vi "Prepare IFDs.vi"(8 "error in (no error)":errorcluster, 11 "TIFF in":refnum<class "TIFF.lvclass">) -> (0 "error out":errorcluster, 3 "TIFF out":refnum<class "TIFF.lvclass">)   [LabVIEW 2018, in "BinaryTIFF.lvlib" / "TIFF.lvclass"]
uses:
  TIFF.lvclass
  TIFF.lvclass/TIFF.ctl
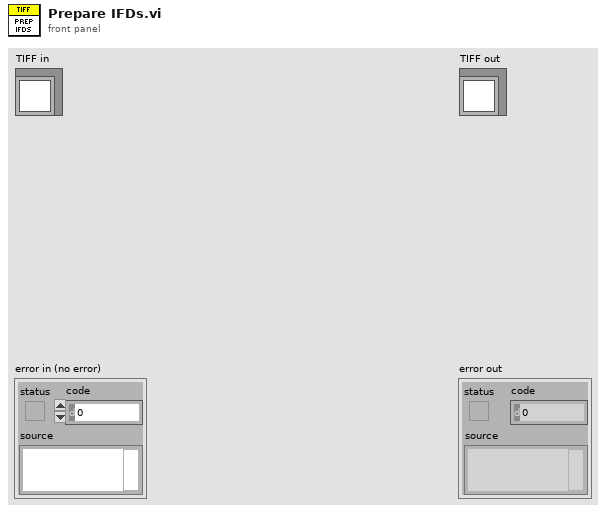
[diagram p1: front panel]
types:
  T1 = cluster{"Offset":u64, "Number of Entries":u64, "IFD Entries":cluster{"Tag":u16, "Data Type":u16, "Number of Elements":u64, "Data":variant}[]}
  T2 = cluster{"Tag":u16, "Data Type":u16, "Number of Elements":u64, "Data":variant}
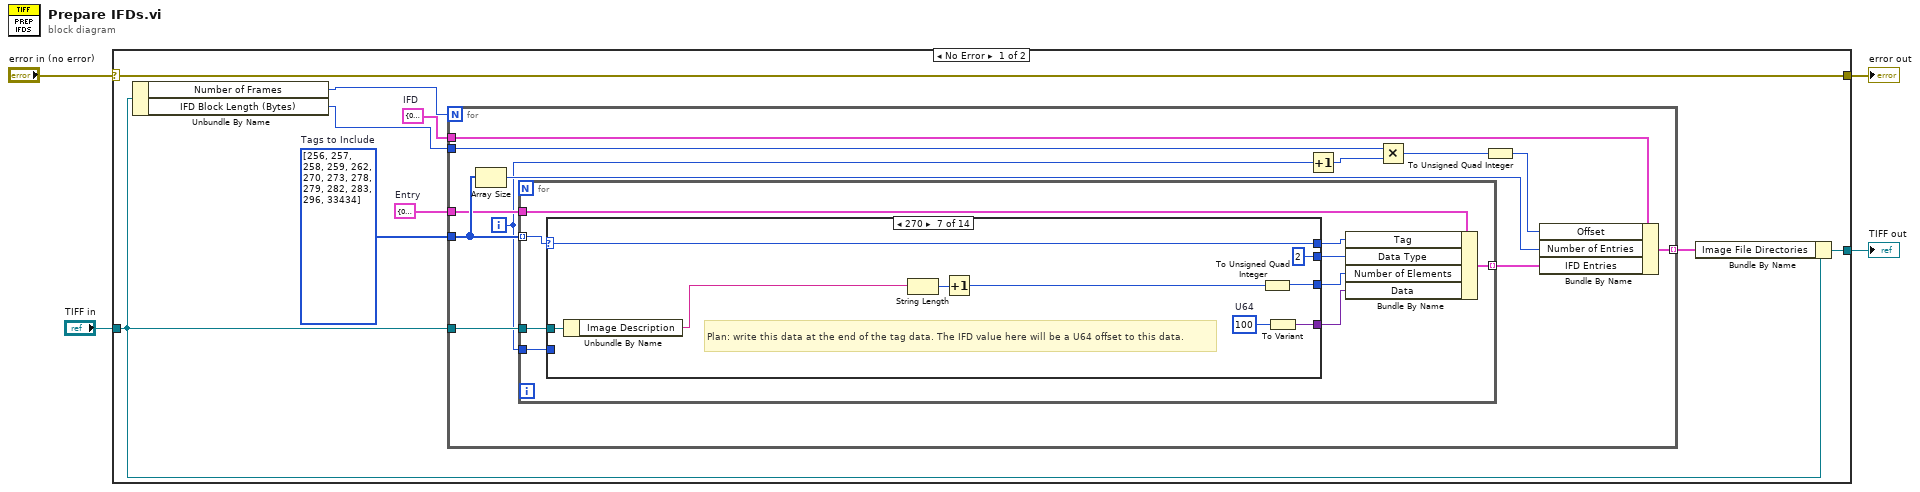
[diagram p0: block diagram]
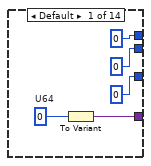
[diagram p2: hidden frame]
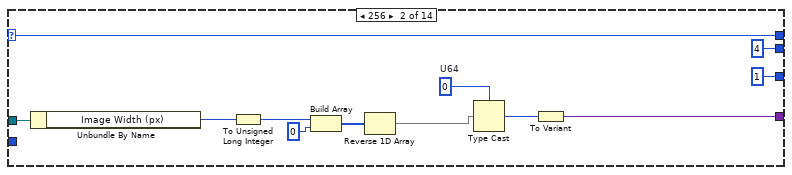
[diagram p3: hidden frame]
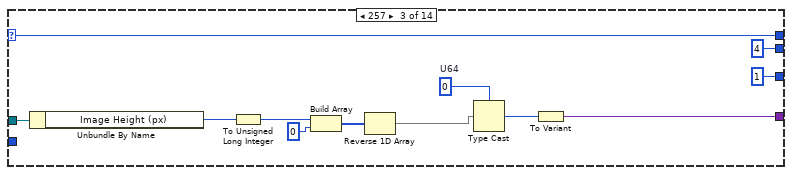
[diagram p4: hidden frame]
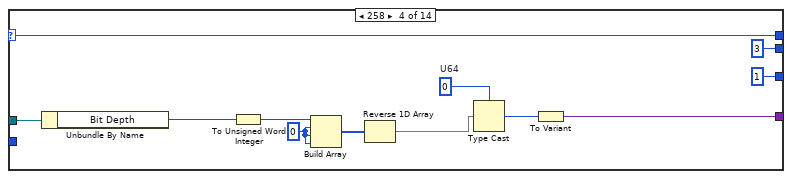
[diagram p5: hidden frame]
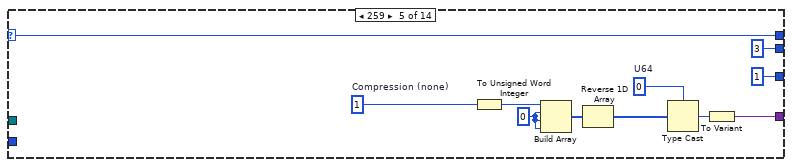
[diagram p6: hidden frame]
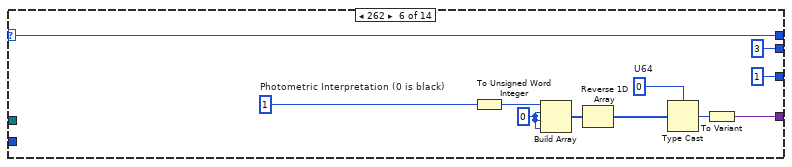
[diagram p7: hidden frame]
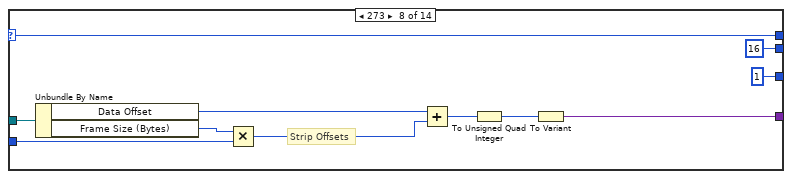
[diagram p8: hidden frame]
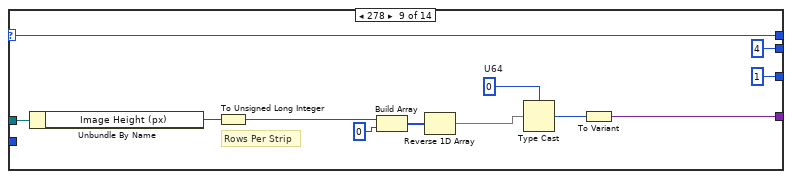
[diagram p9: hidden frame]
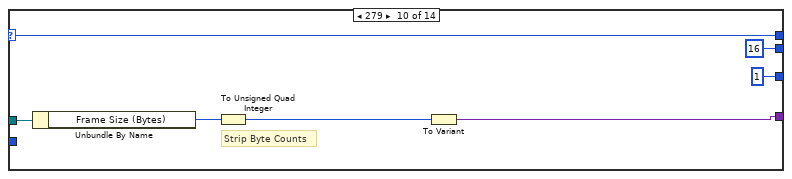
[diagram p10: hidden frame]
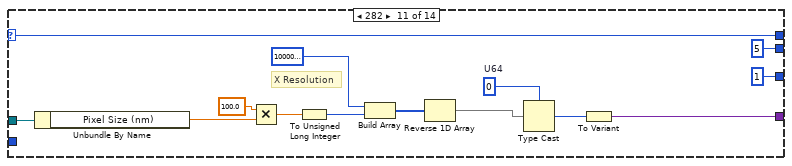
[diagram p11: hidden frame]
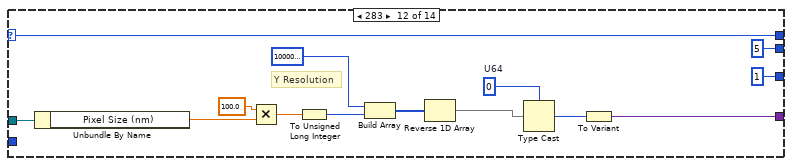
[diagram p12: hidden frame]
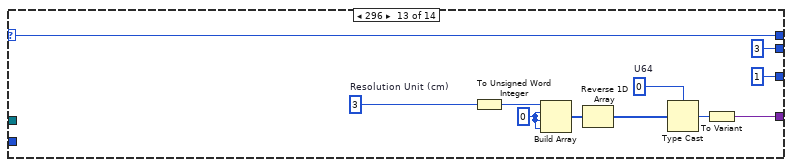
[diagram p13: hidden frame]
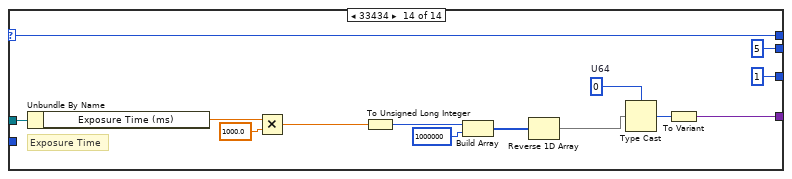
[diagram p14: hidden frame]
diagram:
  n1 = case shown="No Error" "error in (no error)" {
    selector: "error in (no error)" -> [w13 w191]
    tunnel: [w13 w191] -> w3
    tunnel: [w10 w190] -> w1
    tunnel: "TIFF in" -> [w8 w190]
    frame No Error {
      w6 = T1 {"Offset"=0, "Number of Entries"=0, "IFD Entries"=[]}  # IFD
      w7 = T2 {"Tag"=0, "Data Type"=0, "Number of Elements"=0, "Data"=variant}  # Entry
      w11 = u16[] [256, 257, 258, 259, 262, 270, 273, 278, 279, 282, 283, 296, 33434]  # Tags to Include
      n2 = Unbundle By Name(w8) -> ("Number of Frames"=w12:u32, "IFD Block Length (Bytes)"=w9:u32)
      n3 = for {
        N: w12 -> [_]
        tunnel: w11 -> [w22]
        tunnel: w9 -> [w25]
        tunnel: w6 -> [w24]
        tunnel: [w20] -> w5 mode=indexing
        tunnel: w7 -> [w19]
        tunnel: w8 -> [w18]
        i -> [w14]
        n4 = Array Size(array=w22) -> (size(s)=w23:i32)
        n5 = for {
          tunnel: w22 -> [w34] mode=indexing
          tunnel: w18 -> [w33]
          tunnel: w19 -> [w32]
          tunnel: [w31] -> w15 mode=indexing
          tunnel: w14 -> [w26]
          n6 = case shown="270" w34 {
            selector: w34 -> [_ w50 w62 w74 w86 w97 w106 w117 w128 w135 w149 w163 w175 w189]
            tunnel: w33 -> [_ w51 w63 w75 _ _ w104 w114 w129 w136 w150 w164 _ w186]
            tunnel: [u16 0 ("Tag") w50 w62 w74 w86 w97 w106 w117 w128 w135 w149 w163 w175 w189] -> w30
            tunnel: [u16 0 ("Data Type") u16 4 ("Data Type") u16 4 ("Data Type") u16 3 ("Data Type") u16 3 ("Data Type") u16 3 ("Data Type") u16 2 ("Data Type") u16 16 ("Data Type") u16 4 ("Data Type") u16 16 ("Data Type") u16 5 ("Data Type") u16 5 ("Data Type") u16 3 ("Data Type") u16 5 ("Data Type")] -> w29
            tunnel: [u64 0 ("Number of Elements") u64 1 ("Number of Elements") u64 1 ("Number of Elements") u64 1 ("Number of Elements") u64 1 ("Number of Elements") u64 1 ("Number of Elements") w102 u64 1 ("Number of Elements") u64 1 ("Number of Elements") u64 1 ("Number of Elements") u64 1 ("Number of Elements") u64 1 ("Number of Elements") u64 1 ("Number of Elements") u64 1 ("Number of Elements")] -> w28
            tunnel: w26 -> [_ _ _ _ _ _ _ w111 _ _ _ _ _ _]
            tunnel: [w35 w46 w58 w70 w82 w93 w103 w107 w124 w131 w143 w157 w172 w182] -> w27
            frame Default {
              w36 = u64 0  # U64
              n7 = To Variant(anything=w36) -> (Variant=w35:variant)
            }
            frame 256 {
              w43 = u64 0  # U64
              n8 = Unbundle By Name(w51) -> ("Image Width (px)"=w47:u32)
              n9 = To Unsigned Long Integer(number=w47) -> (unsigned 32bit integer=w45:u32)
              n10 = Build Array(w45, u32 0 ("element")) -> (w42:u32[])
              n11 = Reverse 1D Array(array=w42) -> (reversed array=w40:u32[])
              n12 = Type Cast(type=w43, x=w40) -> (*(type *) &x=w41:u64)
              n13 = To Variant(anything=w41) -> (Variant=w46:variant)
            }
            frame 257 {
              w55 = u64 0  # U64
              n14 = Unbundle By Name(w63) -> ("Image Height (px)"=w59:u32)
              n15 = To Unsigned Long Integer(number=w59) -> (unsigned 32bit integer=w56:u32)
              n16 = Build Array(w56, u32 0 ("element")) -> (w54:u32[])
              n17 = Reverse 1D Array(array=w54) -> (reversed array=w52:u32[])
              n18 = Type Cast(type=w55, x=w52) -> (*(type *) &x=w53:u64)
              n19 = To Variant(anything=w53) -> (Variant=w58:variant)
            }
            frame 258 {
              w67 = u64 0  # U64
              w68 = u16 0 ("element")
              n20 = Unbundle By Name(w75) -> ("Bit Depth"=w71:u32)
              n21 = To Unsigned Word Integer(number=w71) -> (unsigned 16bit integer=w69:u16)
              n22 = Build Array(w69, w68, w68, w68) -> (w66:u16[])
              n23 = Reverse 1D Array(array=w66) -> (reversed array=w64:u16[])
              n24 = Type Cast(type=w67, x=w64) -> (*(type *) &x=w65:u64)
              n25 = To Variant(anything=w65) -> (Variant=w70:variant)
            }
            frame 259 {
              w79 = u64 0  # U64
              w81 = u16 0 ("element")
              w83 = u64 1  # Compression (none)
              n26 = To Unsigned Word Integer(number=w83) -> (unsigned 16bit integer=w80:u16)
              n27 = Build Array(w80, w81, w81, w81) -> (w78:u16[])
              n28 = Reverse 1D Array(array=w78) -> (reversed array=w76:u16[])
              n29 = Type Cast(type=w79, x=w76) -> (*(type *) &x=w77:u64)
              n30 = To Variant(anything=w77) -> (Variant=w82:variant)
            }
            frame 262 {
              w90 = u64 0  # U64
              w92 = u16 0 ("element")
              w94 = u64 1  # Photometric Interpretation (0 is black)
              n31 = To Unsigned Word Integer(number=w94) -> (unsigned 16bit integer=w91:u16)
              n32 = Build Array(w91, w92, w92, w92) -> (w89:u16[])
              n33 = Reverse 1D Array(array=w89) -> (reversed array=w87:u16[])
              n34 = Type Cast(type=w90, x=w87) -> (*(type *) &x=w88:u64)
              n35 = To Variant(anything=w88) -> (Variant=w93:variant)
            }
            frame 270 {
              w101 = u64 100  # U64
              # "Plan: write this data at the end of the tag data. The IFD value here will be a U64 offset to this data."
              n36 = Unbundle By Name(w104) -> ("Image Description"=w98:string)
              n37 = String Length(string=w98) -> (length=w100:i32)
              n38 = Increment(x=w100) -> (x+1=w99:i32)
              n39 = To Unsigned Quad Integer(1:w99) -> (0:w102:u64)
              n40 = To Variant(anything=w101) -> (Variant=w103:variant)
            }
            frame 273 {
              # "Strip Offsets"
              n41 = Unbundle By Name(w114) -> ("Data Offset"=w113:u64, "Frame Size (Bytes)"=w112:u64)
              n42 = Multiply(x=w112, y=w111) -> (x*y=w110:u64)
              n43 = Add(x=w113, y=w110) -> (x+y=w109:u64)
              n44 = To Unsigned Quad Integer(1:w109) -> (0:w108:u64)
              n45 = To Variant(anything=w108) -> (Variant=w107:variant)
            }
            frame 278 {
              w121 = u64 0  # U64
              # "Rows Per Strip"
              n46 = Unbundle By Name(w129) -> ("Image Height (px)"=w125:u32)
              n47 = To Unsigned Long Integer(number=w125) -> (unsigned 32bit integer=w122:u32)
              n48 = Build Array(w122, u32 0 ("element")) -> (w120:u32[])
              n49 = Reverse 1D Array(array=w120) -> (reversed array=w118:u32[])
              n50 = Type Cast(type=w121, x=w118) -> (*(type *) &x=w119:u64)
              n51 = To Variant(anything=w119) -> (Variant=w124:variant)
            }
            frame 279 {
              # "Strip Byte Counts"
              n52 = Unbundle By Name(w136) -> ("Frame Size (Bytes)"=w132:u64)
              n53 = To Unsigned Quad Integer(1:w132) -> (0:w130:u64)
              n54 = To Variant(anything=w130) -> (Variant=w131:variant)
            }
            frame 282 {
              w142 = u64 0  # U64
              # "X Resolution"
              n55 = Unbundle By Name(w150) -> ("Pixel Size (nm)"=w146:dbl)
              n56 = Multiply(x=100.0, y=w146) -> (x*y=w144:dbl)
              n57 = To Unsigned Long Integer(number=w144) -> (unsigned 32bit integer=w138:u32)
              n58 = Build Array(u32 1000000000 ("element"), w138) -> (w141:u32[])
              n59 = Reverse 1D Array(array=w141) -> (reversed array=w137:u32[])
              n60 = Type Cast(type=w142, x=w137) -> (*(type *) &x=w140:u64)
              n61 = To Variant(anything=w140) -> (Variant=w143:variant)
            }
            frame 283 {
              w156 = u64 0  # U64
              # "Y Resolution"
              n62 = Unbundle By Name(w164) -> ("Pixel Size (nm)"=w160:dbl)
              n63 = Multiply(x=100.0, y=w160) -> (x*y=w158:dbl)
              n64 = To Unsigned Long Integer(number=w158) -> (unsigned 32bit integer=w153:u32)
              n65 = Build Array(u32 1000000000 ("element"), w153) -> (w155:u32[])
              n66 = Reverse 1D Array(array=w155) -> (reversed array=w151:u32[])
              n67 = Type Cast(type=w156, x=w151) -> (*(type *) &x=w154:u64)
              n68 = To Variant(anything=w154) -> (Variant=w157:variant)
            }
            frame 296 {
              w169 = u64 0  # U64
              w171 = u16 0 ("element")
              w168 = u64 3  # Resolution Unit (cm)
              n69 = To Unsigned Word Integer(number=w168) -> (unsigned 16bit integer=w170:u16)
              n70 = Build Array(w170, w171, w171, w171) -> (w167:u16[])
              n71 = Reverse 1D Array(array=w167) -> (reversed array=w165:u16[])
              n72 = Type Cast(type=w169, x=w165) -> (*(type *) &x=w166:u64)
              n73 = To Variant(anything=w166) -> (Variant=w172:variant)
            }
            frame 33434 {
              w185 = u64 0  # U64
              # "Exposure Time"
              n74 = Unbundle By Name(w186) -> ("Exposure Time (ms)"=w181:dbl)
              n75 = Multiply(x=w181, y=1000.0) -> (x*y=w179:dbl)
              n76 = To Unsigned Long Integer(number=w179) -> (unsigned 32bit integer=w178:u32)
              n77 = Build Array(w178, u32 1000000 ("element")) -> (w184:u32[])
              n78 = Reverse 1D Array(array=w184) -> (reversed array=w176:u32[])
              n79 = Type Cast(type=w185, x=w176) -> (*(type *) &x=w183:u64)
              n80 = To Variant(anything=w183) -> (Variant=w182:variant)
            }
          }
          n81 = Bundle By Name(cluster=w32, "Tag"=w30, "Data Type"=w29, "Number of Elements"=w28, "Data"=w27) -> (w31:T2)
        }
        n82 = Increment(x=w14) -> (x+1=w16:i32)
        n83 = Multiply(x=w25, y=w16) -> (x*y=w17:u32)
        n84 = To Unsigned Quad Integer(1:w17) -> (0:w21:u64)
        n85 = Bundle By Name(cluster=w24, "Offset"=w21, "Number of Entries"=w23, "IFD Entries"=w15) -> (w20:T1)
      }
      n86 = Bundle By Name(cluster=w8, "Image File Directories"=w5) -> (w10:refnum<class "TIFF.lvclass">)
    }
    frame Error {
    }
  }
  "error out" <- w3
  "TIFF out" <- w1
